vi "Unpack for gRPC.vi"(8 "error in":errorcluster, 9 "configuration / results":enum16{"Configuration", "Results"}(ring), 10 "any":T1, 11 "measurement customizations in":refnum<class "Measurement Plugin.lvclass">) -> (0 "error out":errorcluster, 2 "data value":variant, 3 "measurement customizations out":refnum<class "Measurement Plugin.lvclass">)   [LabVIEW 2024, in "Frequency Response (Discrete Sweep).lvlib" / "Measurement Plugin.lvclass"]
uses:
  Measurement Plugin.lvclass
  <vilib>/gRPC/LabVIEW gRPC Library/Shared/Any.ctl
  C:/Program Files/National Instruments/LabVIEW 2024/vi.lib/Plug-In SDKs/Measurements/Measurement Plugin Service/Measurement Plugin Service.lvclass
  Measurement Configuration.ctl
  Measurement Results.ctl
  <vilib>/gRPC/Generated APIs/ni/protobuf/types/RPC Messages/ni_protobuf_types_DoubleXYData.ctl
  a521b266-ce99-437c-923d-067dcf1e07fd.vi
  3ecd018e-d556-4cbc-bc60-c4ba57204520.vi
  <vilib>/gRPC/LabVIEW gRPC Library/Server API/Translate Protobuf Error.vi
  <vilib>/AdvancedString/1D String Array to Delimited String.vi
  <vilib>/gRPC/LabVIEW gRPC Library/Server API/Server/Get Server DLL Path.vi
  Frequency Response (Discrete Sweep).lvlib
  <vilib>/gRPC/Generated APIs/ni/protobuf/types/ni.protobuf.types.lvlib
  <vilib>/Plug-In SDKs/Measurements/Measurement Plugin Service/Measurement Plugin Service.lvclass
  <vilib>/gRPC/LabVIEW gRPC Library/grpc-lvsupport-release.lvlib
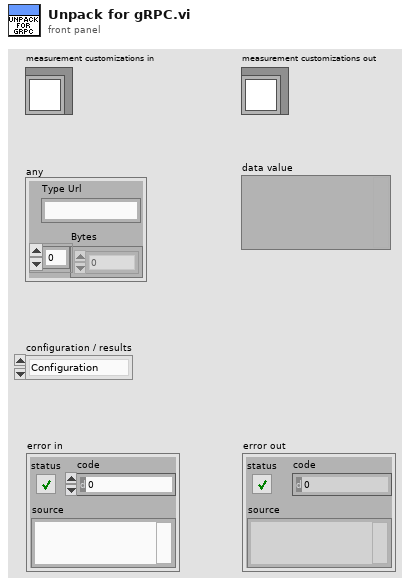
[diagram p1: front panel]
types:
  T1 = typedef "grpc-lvsupport-release.lvlib/Any.ctl" = cluster{"Type Url":string, "Bytes":u8[]}
  T2 = typedef "grpc-lvsupport-release.lvlib/grpcId.ctl" = u64
  T3 = typedef "Frequency Response (Discrete Sweep).lvlib/Measurement Configuration.ctl" = cluster{"sample rate":dbl, "ao stimulus channel":string, "ao range":dbl, "ao terminal configuration":i32, "ai reference channel":string, "ai ref range":dbl, "ai reference terminal configuration":i32, "ai response channel":string, "ai response range":dbl, "ai response terminal configuration":i32, "amplitude":dbl, "start frequency":dbl, "stop frequency":dbl, "number of steps":i32, "profile":enum32{"Linear", "Logarithmic"}, "measurement time":dbl, "measurement cycles":i32}
  T4 = typedef "Frequency Response (Discrete Sweep).lvlib/Measurement Results.ctl" = cluster{"current frequency":dbl, "waveforms file path":string, "reference RMS level":T5, "response RMS level":T5, "FRF magnitude":T5, "FRF phase":T5, "THD":T5, "h2":T5, "h3":T5, "h4":T5, "h5":T5, "THDN":T5}
  T5 = typedef "ni.protobuf.types.lvlib/ni_protobuf_types_DoubleXYData.ctl" = cluster{"x_data":dbl[], "y_data":dbl[]}
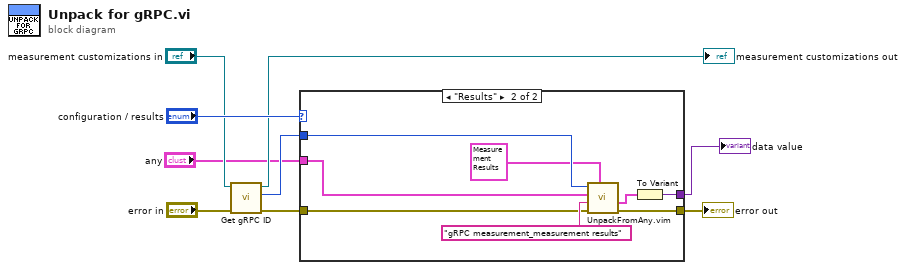
[diagram p0: block diagram]
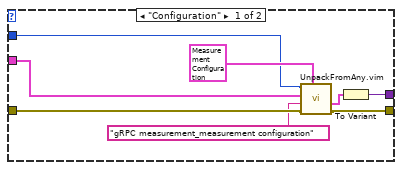
[diagram p2: hidden frame]
diagram:
  n1 = call <vilib>:"Get gRPC ID.vi"("error in"="error in", "measurement plugin service in"="measurement customizations in") -> ("error out"=w6:errorcluster, "gRPC ID"=w3:T2, "measurement plugin service out"=→"measurement customizations out":refnum<class "Measurement Plugin.lvclass">)  [unwired: 7 in]
  n2 = case shown="\"Results\"" "configuration / results" {
    tunnel: w6 -> [w15 w19]
    tunnel: "any" -> [w10 w18]
    tunnel: w3 -> [w12 w22]
    tunnel: [w16 w23] -> w9
    tunnel: [w17 w25] -> w1
    frame "Configuration" {
      n3 = call "UnpackFromAny.vim"("Data Type"=T3 {"sample rate"=1.2, "ao stimulus channel"="Lorem ipsum dolor sit", "ao range"=32.0, "ao terminal configuration"=-32, "ai reference channel"="Dev1/ai0", "ai ref range"=1.0, "ai reference terminal configuration"=1, "ai response channel"="Dev1/ai1", "ai response range"=3.16, "ai response terminal configuration"=-1, "amplitude"=1.4142, "start frequency"=31.25, "stop frequency"=16000.0, "number of steps"=28, "profile"=enum."Logarithmic", "measurement time"=0.001, "measurement cycles"=10} ("Measurement Configuration"), "error in"=w15, "Message Type"="gRPC measurement_measurement configuration", "Any"=w10, "gRPCid in"=w12) -> ("error out"=w16:errorcluster, "Unpacked Value"=w14:T3)  [unwired: 4 in, 1 out]
      n4 = To Variant(anything=w14) -> (Variant=w17:variant)
    }
    frame "Results" {
      n5 = call "UnpackFromAny.vim"("Data Type"=T4 {"current frequency"=0.0, "waveforms file path"="Empty", "reference RMS level"={"x_data"=[], "y_data"=[]}, "response RMS level"={"x_data"=[], "y_data"=[0.0]}, "FRF magnitude"={"x_data"=[0.0], "y_data"=[0.0]}, "FRF phase"={"x_data"=[0.0], "y_data"=[]}, "THD"={"x_data"=[], "y_data"=[]}, "h2"={"x_data"=[], "y_data"=[]}, "h3"={"x_data"=[], "y_data"=[]}, "h4"={"x_data"=[], "y_data"=[]}, "h5"={"x_data"=[], "y_data"=[]}, "THDN"={"x_data"=[], "y_data"=[]}} ("Measurement Results"), "error in"=w19, "Message Type"="gRPC measurement_measurement results", "Any"=w18, "gRPCid in"=w22) -> ("error out"=w23:errorcluster, "Unpacked Value"=w24:T4)  [unwired: 4 in, 1 out]
      n6 = To Variant(anything=w24) -> (Variant=w25:variant)
    }
  }
  "error out" <- w9
  "data value" <- w1
